vi "WriteConfigCuster.vi"(2 "error in (no error)":errorcluster, 3 "Ctrl Reference":refnum<vi>, 4 "ConfigFile (input)":T1) -> (0 "error out":errorcluster, 1 "ConfigFile (output)":T1)   [LabVIEW 2009]
uses:
  <vilib>/Utility/config.llb/Config Data RefNum.ctl
  Write Key (Double).vi
  Write Key (Boolean).vi
  Write Key (Path).vi
  Write Key (String).vi
  <vilib>/Utility/config.llb/NI_LVConfig.lvlib
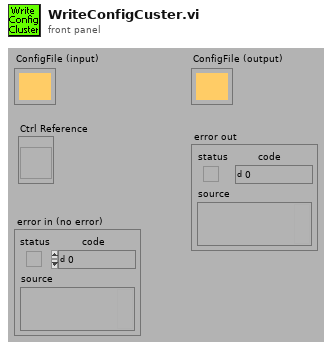
[diagram p1: front panel]
types:
  T1 = typedef "NI_LVConfig.lvlib/Config Data RefNum.ctl" = refnum<k1>
  T2 = typedef "Config Data RefNum" = refnum<k1>
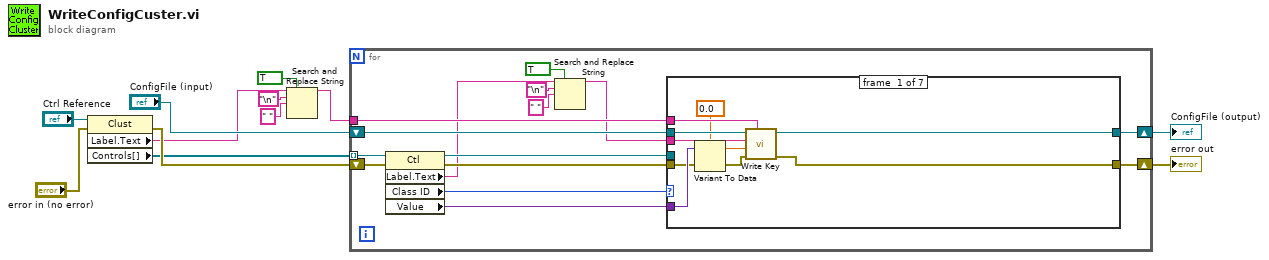
[diagram p0: block diagram]
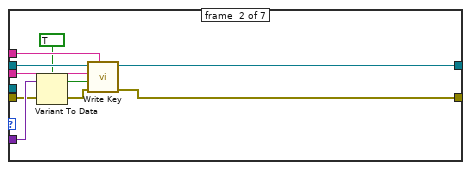
[diagram p2: hidden frame]
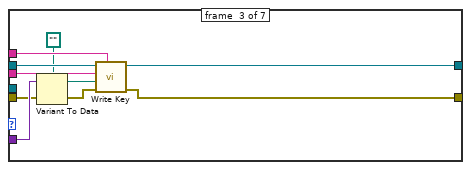
[diagram p3: hidden frame]
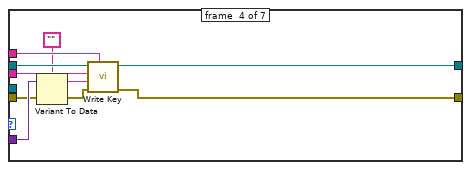
[diagram p4: hidden frame]
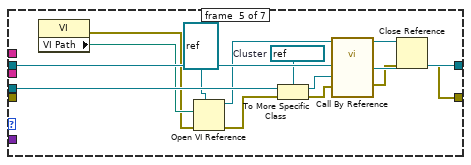
[diagram p5: hidden frame]
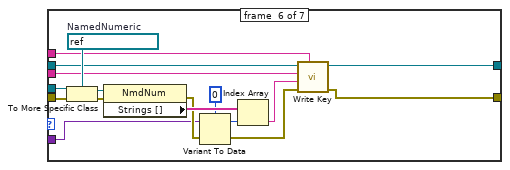
[diagram p6: hidden frame]
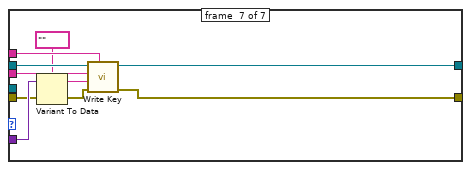
[diagram p7: hidden frame]
diagram:
  n1 = property on="Property Node" class="Clust"(reference="Ctrl Reference", error in="error in (no error)") -> (error out=w8:errorcluster, "Label.Text"=w4:string, "Controls[]"=w6:refnum<vi>[])  [unwired: 1 out]
  n2 = Search and Replace String(replace all?=TRUE ("replace all? (F)"), input string=w4, search string="\n", replace string=" ") -> (result string=w3:string)  [unwired: 4 in, 3 out]
  n3 = for {
    tunnel: w6 -> [w25] mode=indexing
    tunnel: w3 -> [w26]
    shift-right: [w21] -> w9
    shift-left: "ConfigFile (input)" -> [w22]
    shift-right: [w19] -> w12
    shift-left: w8 -> [w20]
    n4 = property on="Property Node" class="Ctl"(reference=w25, error in=w20) -> (reference out=w18:refnum<vi>, error out=w27:errorcluster, "Label.Text"=w14:string, "Class ID"=w24:u32, "Value"=w23:variant)
    n5 = Search and Replace String(replace all?=TRUE ("replace all? (F)"), input string=w14, search string="\n", replace string=" ") -> (result string=w13:string)  [unwired: 4 in, 3 out]
    n6 = case shown="30" w24 {
      tunnel: w22 -> [w37 w47 w57 w67 w81 w86 w108]
      tunnel: w27 -> [w31 w42 w52 w62 _ w97 w103]
      tunnel: w26 -> [w36 w46 w56 w66 _ w85 w107]
      tunnel: w13 -> [w35 w45 w55 w65 _ w84 w106]
      tunnel: w23 -> [w34 w44 w54 w64 _ w89 w105]
      tunnel: [w29 w40 w50 w60 w76 w88 w101] -> w21
      tunnel: [w28 w39 w49 w59 w69 w87 w100] -> w19
      tunnel: w18 -> [_ _ _ _ w79 w98 _]
      frame #0 {
        n7 = Variant To Data(error in=w31, Variant=w34, type=0.0) -> (error out=w30:errorcluster, data=w32:dbl)
        n8 = call-poly "Write Key.vi"("section"=w36, "error in (no error)"=w30, "value"=w32, "key"=w35, "refnum"=w37) -> ("error out"=w28:errorcluster, "refnum out"=w29:T1)  [unwired: 5 in]
      }
      frame #1 {
        n9 = Variant To Data(error in=w42, Variant=w44, type=TRUE) -> (error out=w41:errorcluster, data=w43:bool)
        n10 = call-poly "Write Key.vi"("section"=w46, "error in (no error)"=w41, "value"=w43, "key"=w45, "refnum"=w47) -> ("error out"=w39:errorcluster, "refnum out"=w40:T1)  [unwired: 5 in]
      }
      frame #2 {
        n11 = Variant To Data(error in=w52, Variant=w54, type=path "") -> (error out=w51:errorcluster, data=w53:path)
        n12 = call-poly "Write Key.vi"("section"=w56, "error in (no error)"=w51, "value"=w53, "key"=w55, "refnum"=w57) -> ("error out"=w49:errorcluster, "refnum out"=w50:T1)  [unwired: 5 in]
      }
      frame #3 {
        n13 = Variant To Data(error in=w62, Variant=w64, type="") -> (error out=w61:errorcluster, data=w63:string)
        n14 = call-poly "Write Key.vi"("section"=w66, "error in (no error)"=w61, "value"=w63, "key"=w65, "refnum"=w67) -> ("error out"=w59:errorcluster, "refnum out"=w60:T1)  [unwired: 5 in]
      }
      frame #4 {
        w80 = refnum<vi> refnum  # Cluster
        n15 = property class="VI"() -> (error out=w74:errorcluster, "VI Path"=w75:path)  [unwired: 2 in, 1 out]
        n16 = Open VI Reference(type specifier VI Refnum (for type only)=refnum<vi> refnum, vi path=w75, error in (no error)=w74) -> (vi reference=w73:refnum<vi>, error out=w72:errorcluster)  [unwired: 3 in]
        n17 = To More Specific Class(target class=w80, reference=w79, error in=w72) -> (specific class reference=w78:refnum<vi>, error out=w77:errorcluster)
        n18 = call-by-ref "?"(reference=w73, "error in (no error)"=w77, "Ctrl Reference"=w78, "ConfigFile (input)"=w81) -> (reference out=w70:refnum<vi>, "error out"=w71:errorcluster, "ConfigFile (output)"=w76:T2)  [unwired: 1 in, 1 out]
        n19 = Close Reference(reference=w70, error in (no error)=w71) -> (error out=w69:errorcluster)
      }
      frame #5 {
        w94 = refnum<vi> refnum  # NamedNumeric
        n20 = To More Specific Class(target class=w94, reference=w98, error in=w97) -> (specific class reference=w96:refnum<vi>, error out=w95:errorcluster)
        n21 = property on="Property Node" class="NmdNum"(reference=w96, error in=w95) -> (error out=w91:errorcluster, "Strings []"=w93:string[])  [unwired: 1 out]
        n22 = Variant To Data(error in=w91, Variant=w89, type=0) -> (error out=w83:errorcluster, data=w90:i32)
        n23 = Index Array(array=w93, index=w90) -> (element=w82:string)
        n24 = call-poly "Write Key.vi"("section"=w85, "error in (no error)"=w83, "value"=w82, "key"=w84, "refnum"=w86) -> ("error out"=w87:errorcluster, "refnum out"=w88:T1)  [unwired: 5 in]
      }
      frame #6 {
        n25 = Variant To Data(error in=w103, Variant=w105, type=tag "") -> (error out=w102:errorcluster, data=w104:tag)
        n26 = call-poly "Write Key.vi"("section"=w107, "error in (no error)"=w102, "value"=w104, "key"=w106, "refnum"=w108) -> ("error out"=w100:errorcluster, "refnum out"=w101:T1)  [unwired: 5 in]
      }
    }
  }
  "error out" <- w12
  "ConfigFile (output)" <- w9
